vi "Get_Classical_Lines (subVI).vi"(6 "resolution (# of lines)":u32=800, 8 "error in (no error)":errorcluster, 9 "dB On (F)":bool, 11 "power spectrum":cluster{"f0":dbl, "df":dbl, "Y":dbl[]}) -> (0 "error out":errorcluster, 2 "Unit":string, 3 "spectral lines":cluster{"f0":dbl, "df":dbl, "Y":dbl[]})   [LabVIEW 2023]
doc: "Take the spectral subset (lines) and set the unit string."
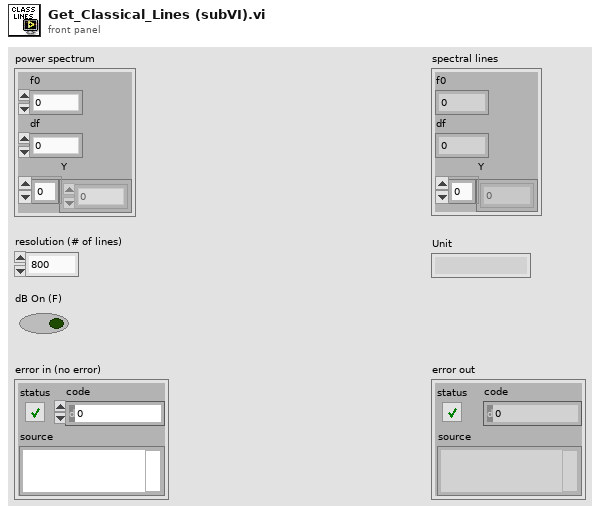
[diagram p1: front panel]
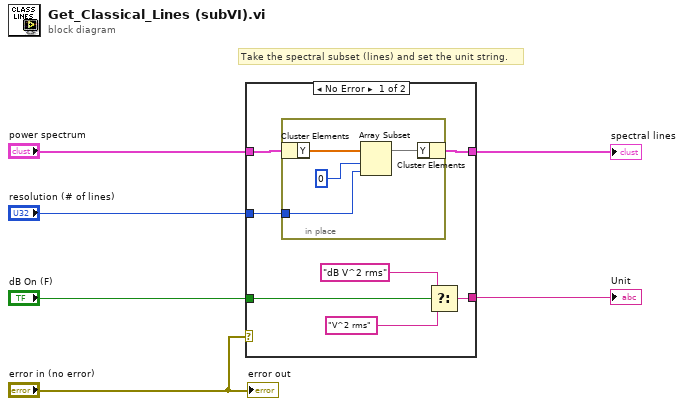
[diagram p0: block diagram]
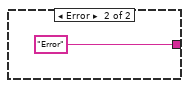
[diagram p2: hidden frame]
diagram:
  # "Take the spectral subset (lines) and set the unit string."
  n1 = case shown="No Error" "error in (no error)" {
    tunnel: "power spectrum" -> [w8 _]
    tunnel: "resolution (# of lines)" -> [w9 _]
    tunnel: "dB On (F)" -> [w11 _]
    tunnel: [w10 "Error" ("Y Scale.Name Label.Text")] -> w4
    tunnel: [w7 _] -> w3
    frame No Error {
      n2 = in-place {
        in-place-border: w9 -> [w16]
        n3 = in-place-cluster #1(w8) -> ("Y"=w15:dbl[])
        n4 = Array Subset(array=w15, index=0 ("Array Index"), length=w16) -> (w14:dbl[])
        n5 = in-place-cluster #1("Y"=w14) -> (w7:cluster{"f0":dbl, "df":dbl, "Y":dbl[]})
      }
      n6 = Select(t="dB V^2 rms" ("Y Scale.Name Label.Text"), s=w11, f="V^2 rms" ("Y Scale.Name Label.Text")) -> (s? t:f=w10:string)
    }
    frame Error {
    }
  }
  "spectral lines" <- w3
  "Unit" <- w4
  "error out" <- "error in (no error)"
